vi "Boiler.vi"() -> ()   [LabVIEW 2013]
uses:
  Controls/Boiler Controls.ctl
  Controls/Boiler Simulation Controls.ctl
  Controls/Boiler Status Indicators.ctl
  Controls/Boiler Application Controls.ctl
  Controls/Boiler States.ctl
  Controls/Purge States.ctl
panel:
  in  "Stop":T1
  out "Boiler Status Indicators":T2 {"Time Count" format="%.2g"}
  in  "Boiler Simulation Controls":T3 {"Flame Sensor Value (%)" min=0.0 max=100.0 scale=0.0..100.0}
  in  "Boiler Controls":T4 {"Fuel Valve Position" min=0.0 max=100.0 scale=0.0..100.0 scale format="%.2f"}
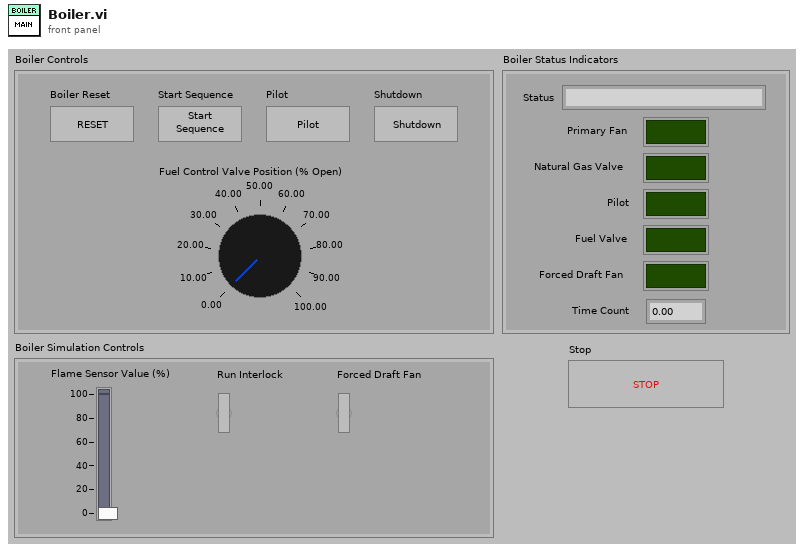
[diagram p1: front panel]
types:
  T1 = typedef "Boiler Application Controls.ctl" = bool
  T2 = typedef "Boiler Status Indicators.ctl" = cluster{"Status":string, "Primary Fan":bool, "Natural Gas Valve":bool, "Pilot":bool, "Fuel Valve":bool, "Forced Draft Fan":bool, "Time Count":dbl}
  T3 = typedef "Boiler Simulation Controls.ctl" = cluster{"Flame Sensor Value (%)":dbl, "Run Interlock":bool, "Forced Draft Fan":bool}
  T4 = typedef "Boiler Controls.ctl" = cluster{"Boiler Reset":bool, "Start Sequence":bool, "Pilot":bool, "Shutdown":bool, "Fuel Valve Position":dbl}
  T5 = typedef "Purge States.ctl" = enum16{"Pre-Purge", "Purge"}
  T6 = typedef "Boiler States.ctl" = enum16{"Initialize", "Main", "Reset Timeout", "Run Cont.", "Shutdown", "Stop"}
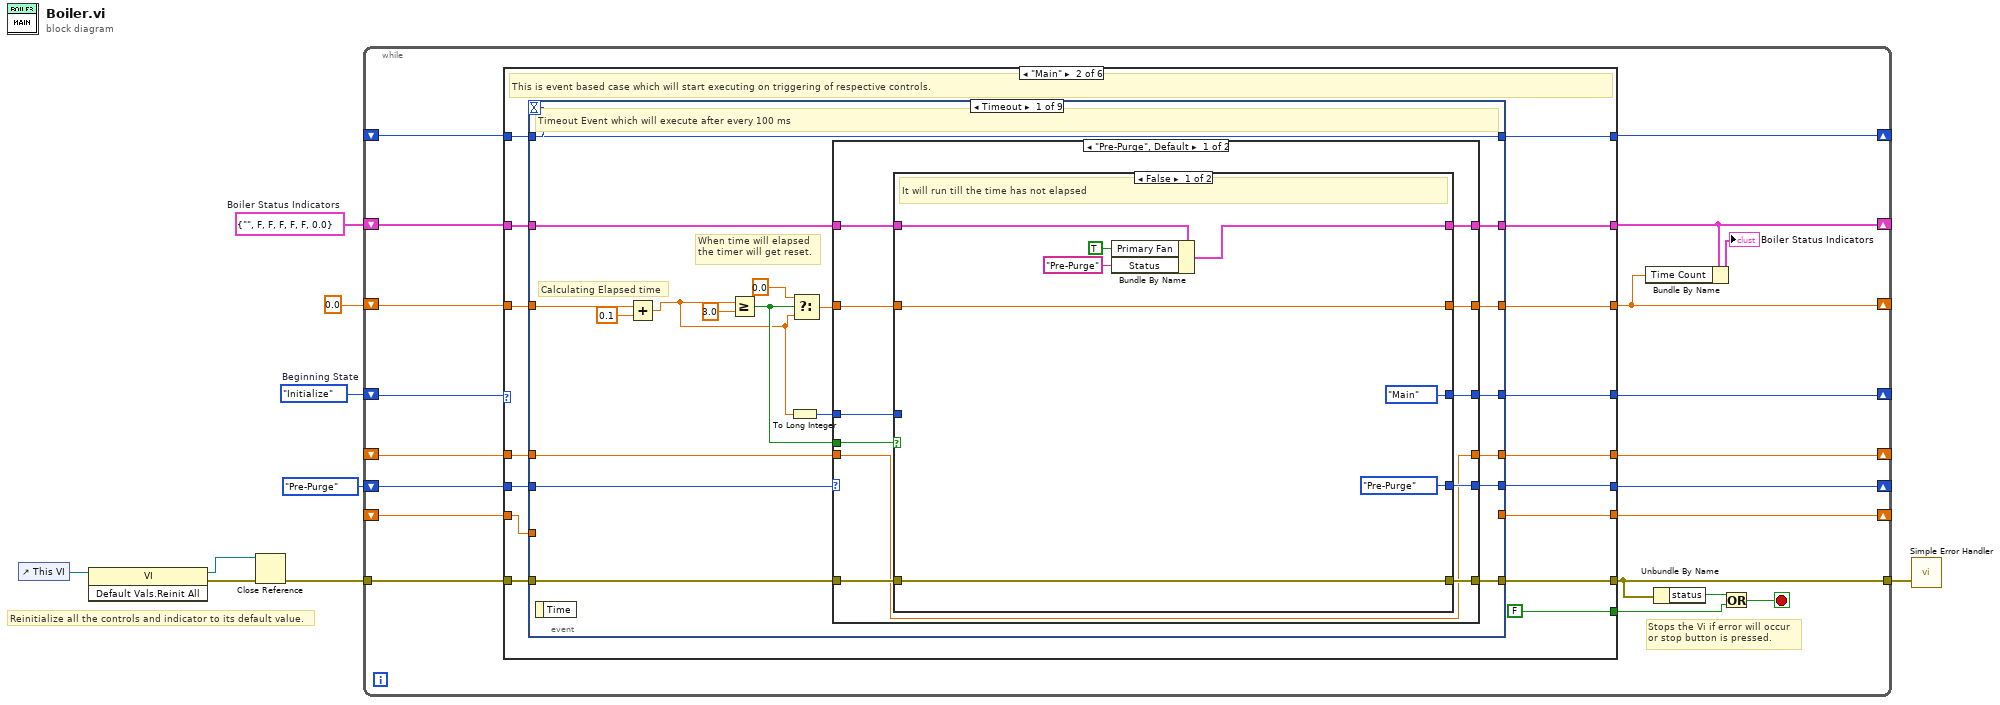
[diagram p0: block diagram]
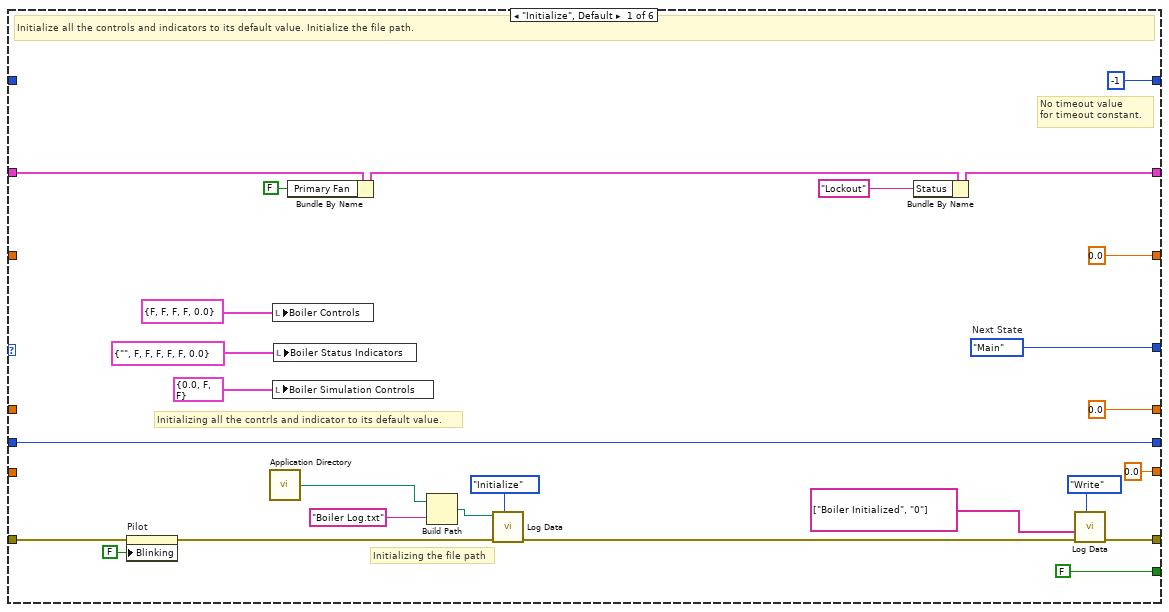
[diagram p2: hidden frame]
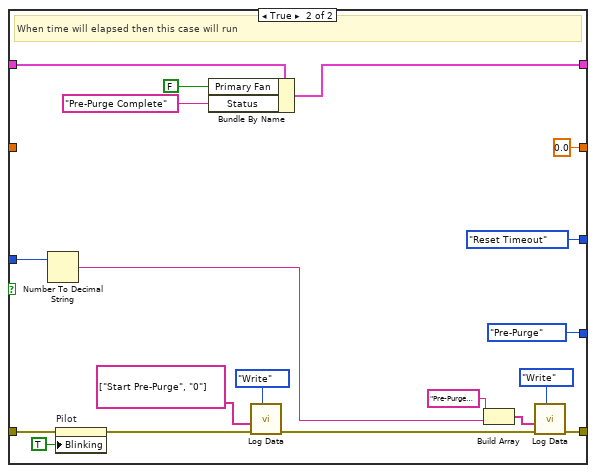
[diagram p3: hidden frame]
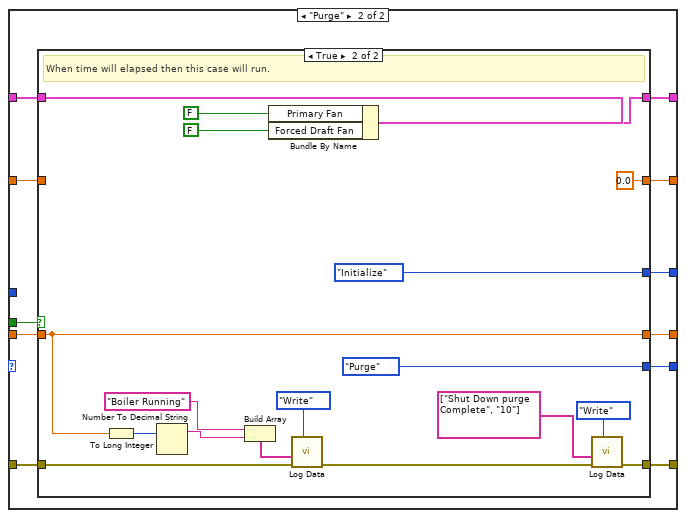
[diagram p4: hidden frame]
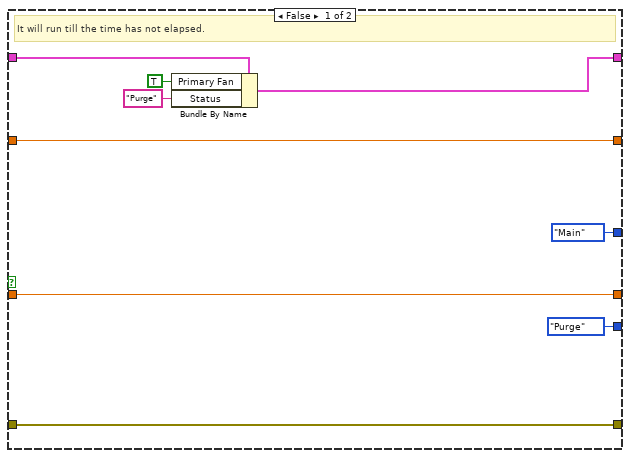
[diagram p5: hidden frame]
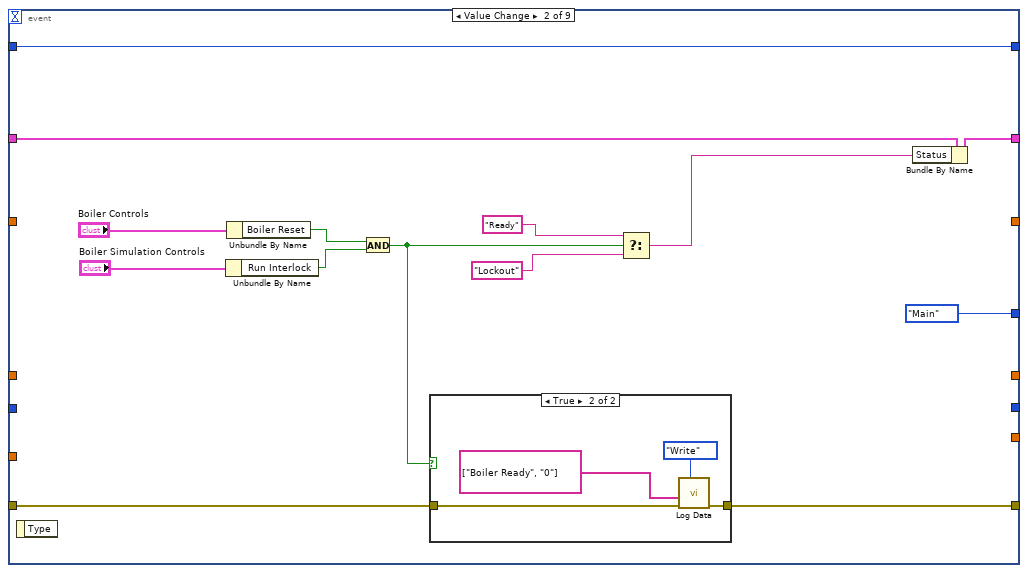
[diagram p6: hidden frame]
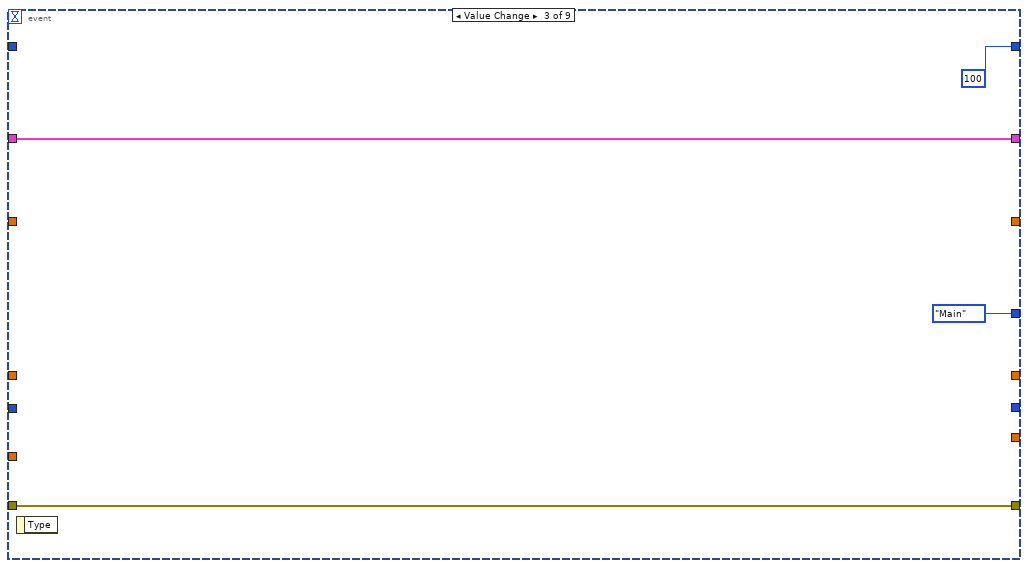
[diagram p8: hidden frame]
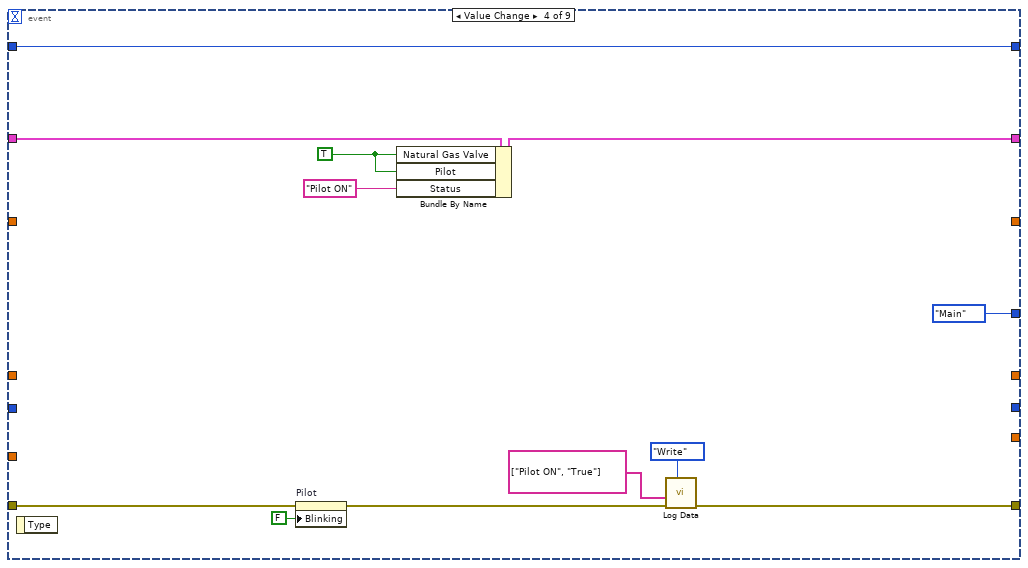
[diagram p9: hidden frame]
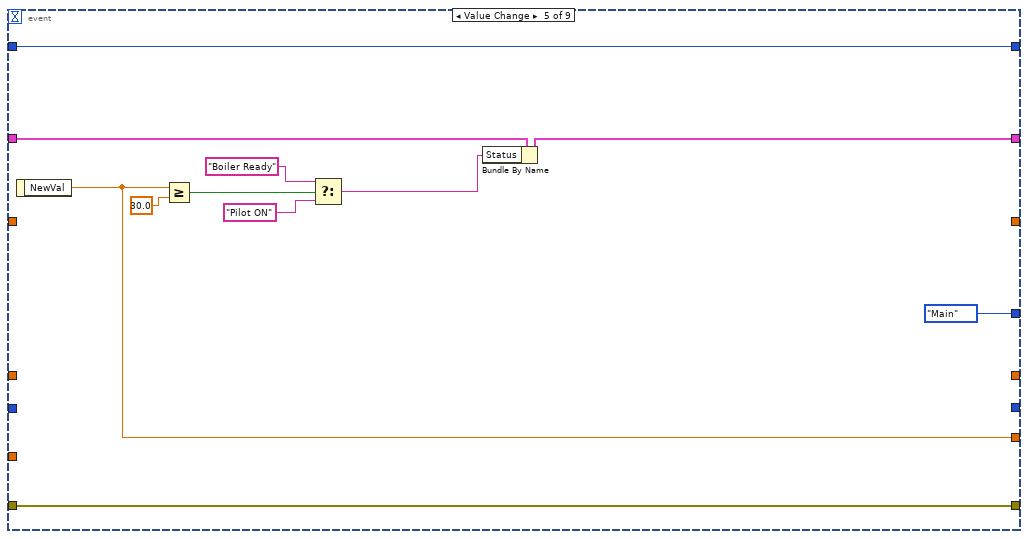
[diagram p10: hidden frame]
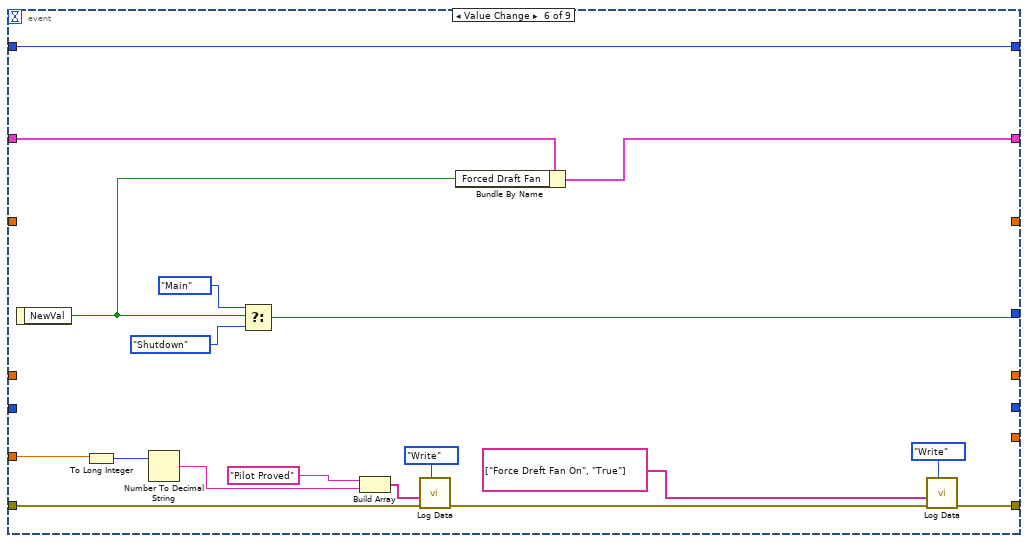
[diagram p11: hidden frame]
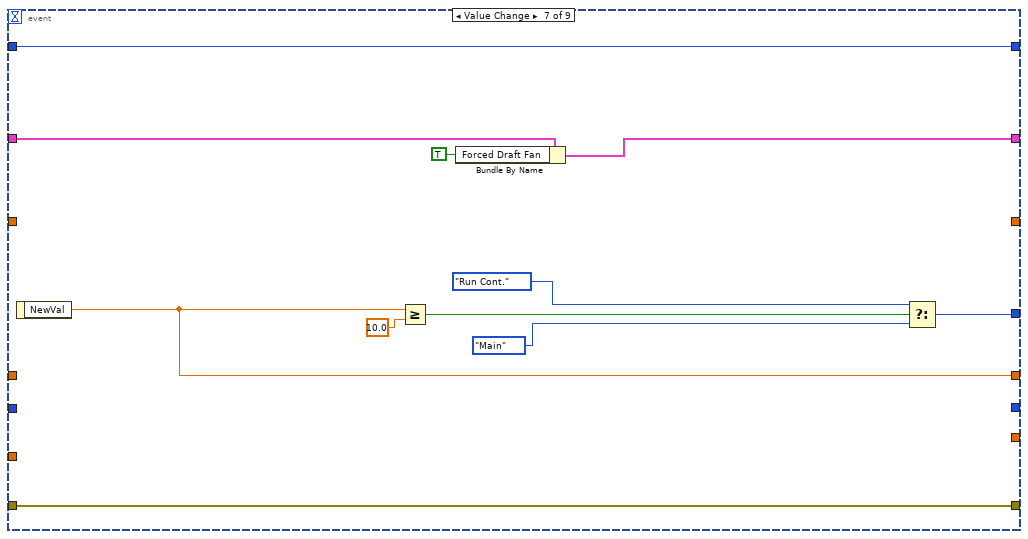
[diagram p12: hidden frame]
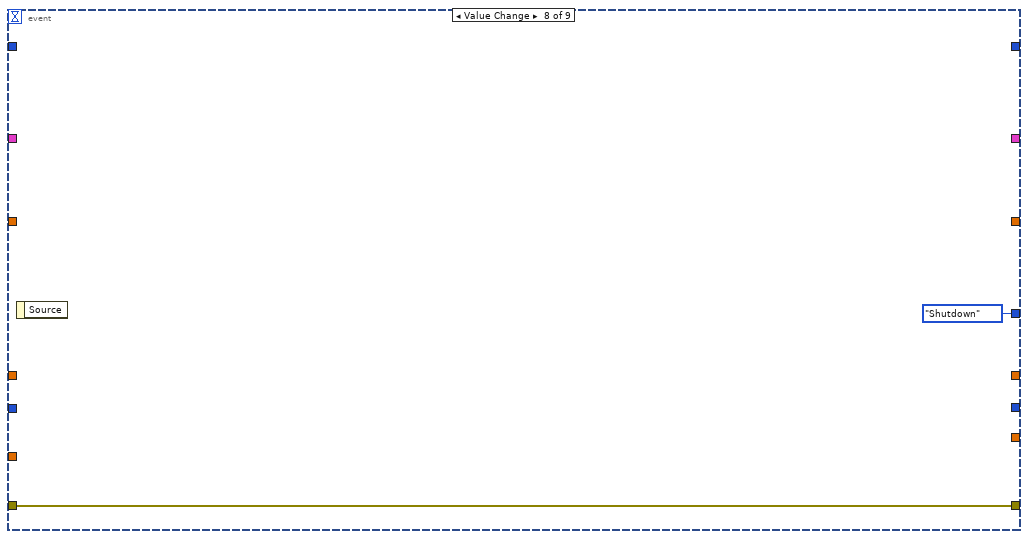
[diagram p13: hidden frame]
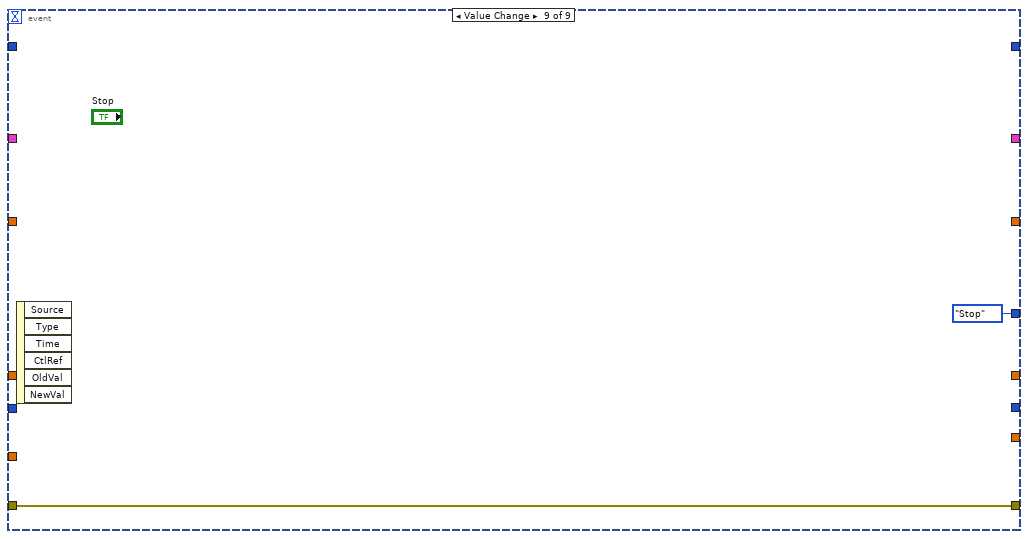
[diagram p14: hidden frame]
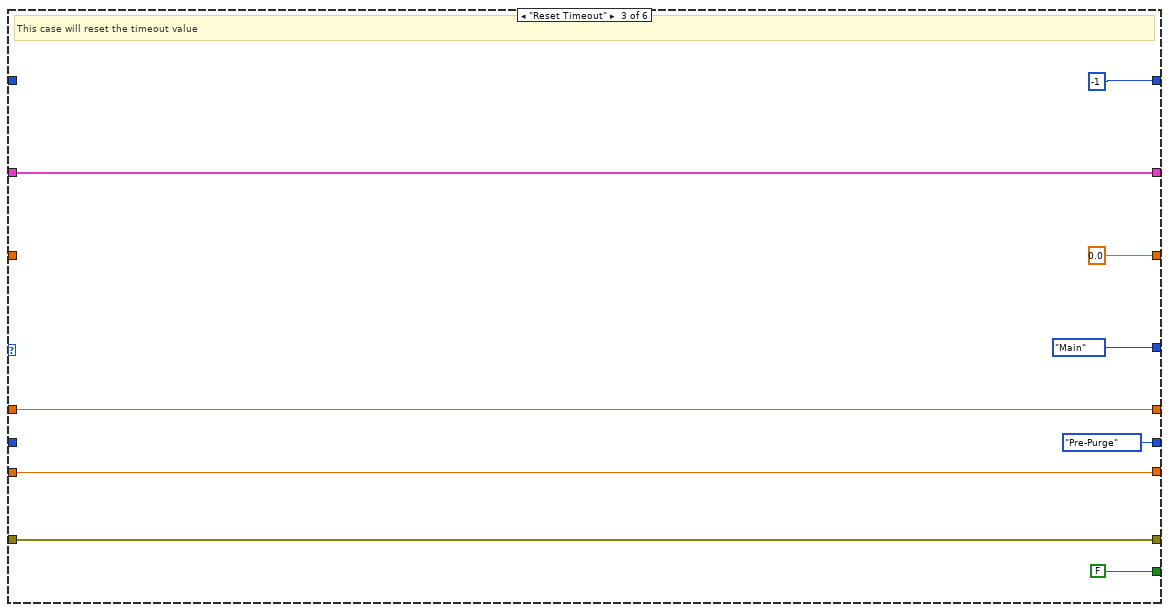
[diagram p15: hidden frame]
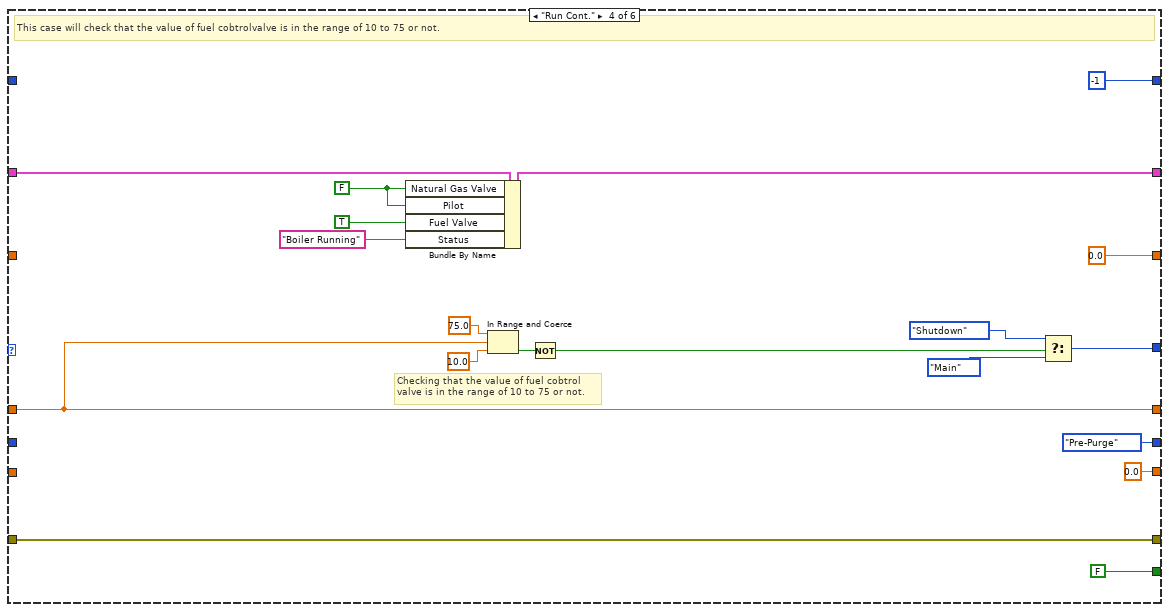
[diagram p16: hidden frame]
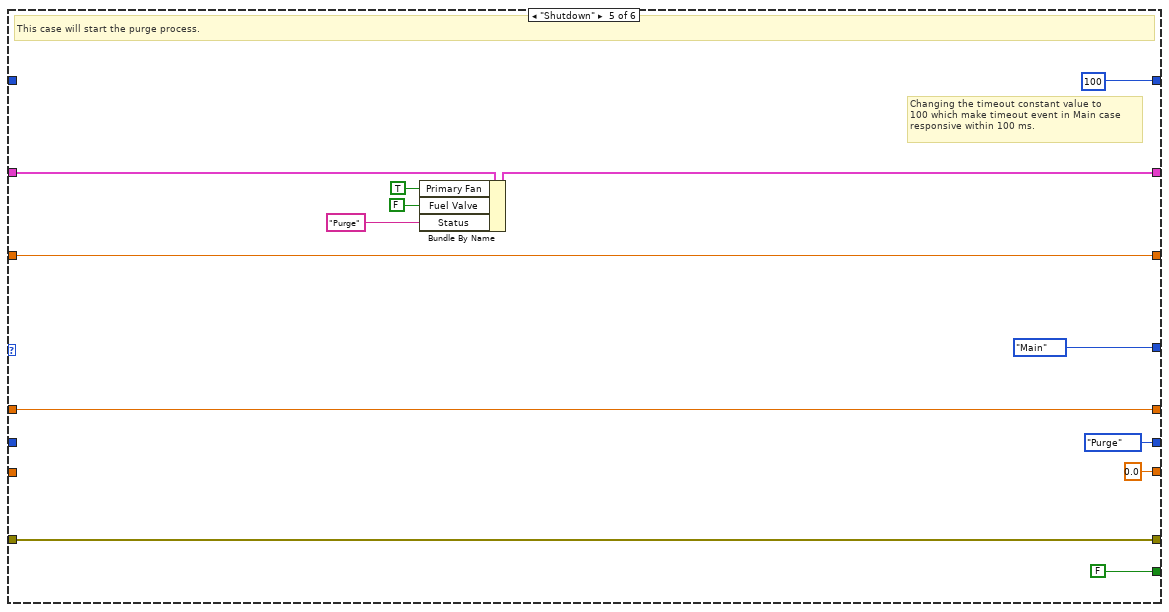
[diagram p17: hidden frame]
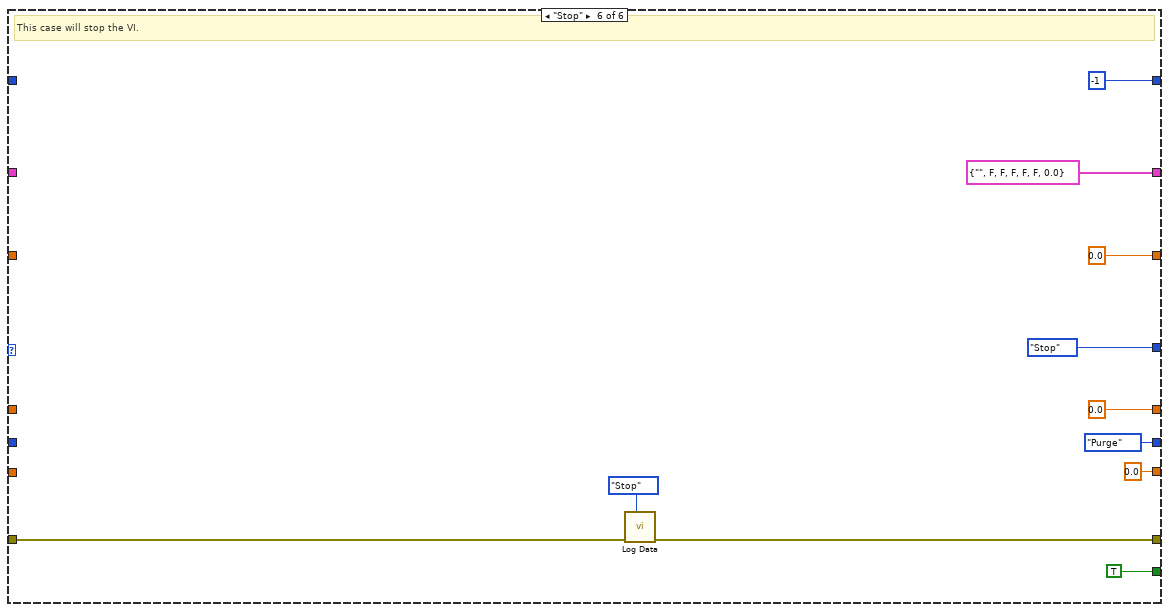
[diagram p18: hidden frame]
diagram:
  w3 = T2 {"Status"="", "Primary Fan"=FALSE, "Natural Gas Valve"=FALSE, "Pilot"=FALSE, "Fuel Valve"=FALSE, "Forced Draft Fan"=FALSE, "Time Count"=0.0}  # Boiler Status Indicators
  w9 = Boiler_States."Initialize"  # Beginning State
  # "Reinitialize all the controls and indicator to its default value."
  n1 = control-ref of="This VI"() -> (w8:refnum<vi>)
  n2 = invoke class="VI" method="Default Vals.Reinit All"(reference=w8) -> (reference out=w6:refnum<vi>, error out=w7:errorcluster)  [unwired: 2 in, 1 out]
  n3 = Close Reference(reference=w6, error in (no error)=w7) -> (error out=w5:errorcluster)
  n4 = while {
    shift-right: [w28] -> _
    shift-left: w9 -> [w29]
    tunnel: w5 -> [w27]
    tunnel: [w26] -> w4
    shift-right: [w22] -> _
    shift-left: _ -> [w19]
    shift-right: [w20] -> _
    shift-left: w3 -> [w21]
    shift-right: [w16] -> _
    shift-left: 0.0 -> [w18]
    shift-right: [w15] -> _
    shift-left: _ -> [w14]
    shift-right: [w12] -> _
    shift-left: Purge_States."Pre-Purge" -> [w13]
    shift-right: [w11] -> _
    shift-left: _ -> [w10]
    stop <- w25 stop-if-true
    # "Stops the Vi if error will occur \nor stop button is pressed."
    n5 = case shown="\"Main\"" w29 {
      tunnel: [w55 w62 Boiler_States."Main" ("Next State") w261 Boiler_States."Main" ("Next State") Boiler_States."Stop" ("Next State")] -> w28
      tunnel: w27 -> [w45 w70 w247 w271 w276 w290]
      tunnel: [w33 w69 w247 w271 w276 w289] -> w26
      tunnel: [FALSE FALSE FALSE FALSE FALSE TRUE] -> w23
      tunnel: [-1 w68 -1 -1 100 -1] -> w22
      tunnel: [w47 w66 w253 w269 w284 T2 {"Status"="", "Primary Fan"=FALSE, "Natural Gas Valve"=FALSE, "Pilot"=FALSE, "Fuel Valve"=FALSE, "Forced Draft Fan"=FALSE, "Time Count"=0.0} ("Boiler Status Indicators")] -> w20
      tunnel: w21 -> [w50 w67 w253 w273 w286 _]
      tunnel: w19 -> [_ w65 _ _ _ _]
      tunnel: w18 -> [_ w64 _ _ w277 _]
      tunnel: [0.0 ("t") w63 0.0 ("t") 0.0 ("t") w277 0.0 ("t")] -> w16
      tunnel: [0.0 ("NewVal") w61 w249 w260 w274 0.0 ("NewVal")] -> w15
      tunnel: w14 -> [_ w56 w249 w260 w274 _]
      tunnel: w13 -> [w42 w60 _ _ _ _]
      tunnel: [w42 w59 Purge_States."Pre-Purge" Purge_States."Pre-Purge" Purge_States."Purge" Purge_States."Purge"] -> w12
      tunnel: [0.0 ("NewVal") w58 w246 0.0 ("NewVal") 0.0 ("NewVal") 0.0 ("NewVal")] -> w11
      tunnel: w10 -> [_ w57 w246 _ _ _]
      frame "Initialize", Default {
        w55 = Boiler_States."Main"  # Next State
        # "No timeout value \nfor timeout constant."
        # "Initializing the file path"
        # "Initializing all the contrls and indicator to its default value."
        # "Initialize all the controls and indicators to its default value. Initialize the file path."
        n6 = property on="Pilot" class="Bool (strict)"(error in=w45, "Blinking"=FALSE) -> (error out=w39:errorcluster)  [unwired: 1 in, 1 out]
        n7 = call <vilib>:"Application Directory.vi"() -> ("Application Directory"=w37:path)
        n8 = local write "Boiler Controls"(T4 {"Boiler Reset"=FALSE, "Start Sequence"=FALSE, "Pilot"=FALSE, "Shutdown"=FALSE, "Fuel Valve Position"=0.0} ("Boiler Controls")) -> ()
        n9 = local write "Boiler Simulation Controls"(T3 {"Flame Sensor Value (%)"=0.0, "Run Interlock"=FALSE, "Forced Draft Fan"=FALSE} ("Boiler Simulation Controls")) -> ()
        n10 = local write "Boiler Status Indicators"(T2 {"Status"="", "Primary Fan"=FALSE, "Natural Gas Valve"=FALSE, "Pilot"=FALSE, "Fuel Valve"=FALSE, "Forced Draft Fan"=FALSE, "Time Count"=0.0} ("Boiler Status Indicators")) -> ()
        n11 = Bundle By Name(cluster=w50, "Primary Fan"=FALSE) -> (w41:T2)
        n12 = Build Path(base path=w37, name or relative path="Boiler Log.txt") -> (appended path=w36:path)
        n13 = call "Log Data.vi"("Command"=enum16{"Initialize", "Write", "Stop"}."Initialize", "error in (no error)"=w39, "file path"=w36) -> ("error out"=w34:errorcluster)  [unwired: 8 in]
        n14 = Bundle By Name(cluster=w41, "Status"="Lockout") -> (w47:T2)
        n15 = call "Log Data.vi"("Command"=enum16{"Initialize", "Write", "Stop"}."Write", "error in (no error)"=w34, "Event Data"=string[] ["Boiler Initialized", "0"]) -> ("error out"=w33:errorcluster)  [unwired: 8 in]
      }
      frame "Main" {
        # "This is event based case which will start executing on triggering of respective controls."
        n16 = event shown="[0] Timeout" {
          selector: _ -> [_ _ _ _ _ _ _ _ _]
          dyn-events: _ -> [_ _ _ _ _ _ _ _ _]
          timeout: w65 -> [_ _ _ _ _ _ _ _ _]
          tunnel: w70 -> [w82 w168 w189 w198 w202 w217 w232 w242 w245]
          tunnel: [w81 w167 w189 w192 w202 w223 w232 w242 w245] -> w69
          tunnel: [w86 w172 100 w199 w204 w228 w238 _ _] -> w68
          tunnel: w67 -> [w80 w175 w188 w201 w210 w229 w240 _ _]
          tunnel: [w79 w174 w188 w196 w209 w230 w241 _ _] -> w66
          tunnel: w65 -> [w86 w172 _ w199 w204 w228 w238 _ _]
          tunnel: [w84 _ _ _ _ _ _ _ _] -> w63
          tunnel: w64 -> [w90 _ _ _ _ _ _ _ _]
          tunnel: [w78 Boiler_States."Main" ("Next State") Boiler_States."Main" ("Next State") Boiler_States."Main" ("Next State") Boiler_States."Main" ("Next State") w225 w233 Boiler_States."Shutdown" ("Next State") Boiler_States."Stop" ("Next State")] -> w62
          tunnel: [w72 _ _ _ _ _ w231 _ _] -> w61
          tunnel: w60 -> [w77 _ _ _ _ _ _ _ _]
          tunnel: [w76 _ _ _ _ _ _ _ _] -> w59
          tunnel: [_ _ _ _ w203 _ _ _ _] -> w58
          tunnel: w57 -> [_ _ _ _ _ w214 _ _ _]
          tunnel: w56 -> [w73 _ _ _ _ _ _ _ _]
          event Timeout {
            # "When time will elapsed \nthe timer will get reset."
            # "Calculating Elapsed time"
            # "Timeout Event which will execute after every 100 ms"
            n17 = event-data() -> ()  [unwired: 1 in, 1 out]
            n18 = Add(x=w90, y=0.1) -> (x+y=w75:dbl)
            n19 = Greater Or Equal?(x=w75, y=3.0) -> (x >= y?=w85:bool)
            n20 = To Long Integer(number=w75) -> (32bit integer=w74:i32)
            n21 = Select(t=0.0, s=w85, f=w75) -> (s? t:f=w83:dbl)
            n22 = case shown="\"Pre-Purge\", Default" w77 {
              tunnel: w85 -> [w101 w139]
              tunnel: [w100 w138] -> w84
              tunnel: w83 -> [w99 w137]
              tunnel: w82 -> [w98 w136]
              tunnel: [w97 w135] -> w81
              tunnel: w80 -> [w96 w134]
              tunnel: [w95 w133] -> w79
              tunnel: [w94 w132] -> w78
              tunnel: [w93 w131] -> w76
              tunnel: w74 -> [w92 _]
              tunnel: w73 -> [w91 w130]
              tunnel: [w91 w129] -> w72
              frame "Pre-Purge", Default {
                n23 = case shown="False" w101 {
                  tunnel: [w109 0.0 ("t")] -> w100
                  tunnel: w99 -> [w109 _]
                  tunnel: w98 -> [w102 w127]
                  tunnel: [w102 w119] -> w97
                  tunnel: w96 -> [w106 w123]
                  tunnel: [w105 w122] -> w95
                  tunnel: [Boiler_States."Main" ("Next State") Boiler_States."Reset Timeout" ("Next State")] -> w94
                  tunnel: [Purge_States."Pre-Purge" Purge_States."Pre-Purge"] -> w93
                  tunnel: w92 -> [_ w118]
                  frame False {
                    # "It will run till the time has not elapsed"
                    n24 = Bundle By Name(cluster=w106, "Primary Fan"=TRUE, "Status"="Pre-Purge") -> (w105:T2)
                  }
                  frame True {
                    # "When time will elapsed then this case will run"
                    n25 = Number To Decimal String(number=w118) -> (decimal integer string=w117:string)  [unwired: 1 in]
                    n26 = property on="Pilot" class="Bool (strict)"(error in=w127, "Blinking"=TRUE) -> (error out=w112:errorcluster)  [unwired: 1 in, 1 out]
                    n27 = Bundle By Name(cluster=w123, "Primary Fan"=FALSE, "Status"="Pre-Purge Complete") -> (w122:T2)
                    n28 = call "Log Data.vi"("Command"=enum16{"Initialize", "Write", "Stop"}."Write", "error in (no error)"=w112, "Event Data"=string[] ["Start Pre-Purge", "0"]) -> ("error out"=w111:errorcluster)  [unwired: 8 in]
                    n29 = Build Array("Pre-Purge Complete", w117) -> (w114:string[])
                    n30 = call "Log Data.vi"("Command"=enum16{"Initialize", "Write", "Stop"}."Write", "error in (no error)"=w111, "Event Data"=w114) -> ("error out"=w119:errorcluster)  [unwired: 8 in]
                  }
                }
              }
              frame "Purge" {
                # "Pre-Purge Case"
                n31 = case shown="True" w139 {
                  tunnel: [w148 0.0 ("t")] -> w138
                  tunnel: w137 -> [w148 _]
                  tunnel: w136 -> [w147 w151]
                  tunnel: [w147 w157] -> w135
                  tunnel: w134 -> [w144 w165]
                  tunnel: [w143 w162] -> w133
                  tunnel: [Boiler_States."Main" ("Next State") Boiler_States."Initialize" ("Next State")] -> w132
                  tunnel: [Purge_States."Purge" Purge_States."Purge"] -> w131
                  tunnel: w130 -> [w140 w149]
                  tunnel: [w140 w149] -> w129
                  frame False {
                    # "It will run till the time has not elapsed."
                    n32 = Bundle By Name(cluster=w144, "Primary Fan"=TRUE, "Status"="Purge") -> (w143:T2)
                  }
                  frame True {
                    # "When time will elapsed then this case will run."
                    n33 = To Long Integer(number=w149) -> (32bit integer=w156:i32)
                    n34 = Number To Decimal String(number=w156) -> (decimal integer string=w155:string)  [unwired: 1 in]
                    n35 = Build Array("Boiler Running", w155) -> (w153:string[])
                    n36 = Bundle By Name(cluster=w165, "Primary Fan"=FALSE, "Forced Draft Fan"=FALSE) -> (w162:T2)
                    n37 = call "Log Data.vi"("Command"=enum16{"Initialize", "Write", "Stop"}."Write", "error in (no error)"=w151, "Event Data"=w153) -> ("error out"=w150:errorcluster)  [unwired: 8 in]
                    n38 = call "Log Data.vi"("Command"=enum16{"Initialize", "Write", "Stop"}."Write", "error in (no error)"=w150, "Event Data"=string[] ["Shut Down purge Complete", "10"]) -> ("error out"=w157:errorcluster)  [unwired: 8 in]
                  }
                }
              }
            }
          }
          event Value Change {
            n39 = event-data() -> ()  [unwired: 1 in, 1 out]
            n40 = Unbundle By Name("Boiler Simulation Controls") -> ("Run Interlock"=w171:bool)
            n41 = Unbundle By Name("Boiler Controls") -> ("Boiler Reset"=w178:bool)
            n42 = And(x=w178, y=w171) -> (x .and. y?=w169:bool)
            n43 = case shown="True" w169 {
              tunnel: w168 -> [w181 w185]
              tunnel: [w181 w184] -> w167
              frame False {
              }
              frame True {
                n44 = call "Log Data.vi"("Command"=enum16{"Initialize", "Write", "Stop"}."Write", "error in (no error)"=w185, "Event Data"=string[] ["Boiler Ready", "0"]) -> ("error out"=w184:errorcluster)  [unwired: 8 in]
              }
            }
            n45 = Select(t="Ready", s=w169, f="Lockout") -> (s? t:f=w173:string)
            n46 = Bundle By Name(cluster=w175, "Status"=w173) -> (w174:T2)
          }
          event Value Change {
            n47 = event-data() -> ()  [unwired: 1 in, 1 out]
          }
          event Value Change {
            w195 = TRUE ("Natural Gas Valve")
            n48 = event-data() -> ()  [unwired: 1 in, 1 out]
            n49 = property on="Pilot" class="Bool (strict)"(error in=w198, "Blinking"=FALSE) -> (error out=w193:errorcluster)  [unwired: 1 in, 1 out]
            n50 = Bundle By Name(cluster=w201, "Natural Gas Valve"=w195, "Pilot"=w195, "Status"="Pilot ON") -> (w196:T2)
            n51 = call "Log Data.vi"("Command"=enum16{"Initialize", "Write", "Stop"}."Write", "error in (no error)"=w193, "Event Data"=string[] ["Pilot ON", "True"]) -> ("error out"=w192:errorcluster)  [unwired: 8 in]
          }
          event Value Change {
            n52 = event-data() -> ("NewVal"=w203:dbl)  [unwired: 1 in]
            n53 = Greater Or Equal?(x=w203, y=30.0) -> (x >= y?=w211:bool)
            n54 = Select(t="Boiler Ready", s=w211, f="Pilot ON") -> (s? t:f=w206:string)
            n55 = Bundle By Name(cluster=w210, "Status"=w206) -> (w209:T2)
          }
          event Value Change {
            n56 = event-data() -> ("NewVal"=w224:bool)  [unwired: 1 in]
            n57 = To Long Integer(number=w214) -> (32bit integer=w218:i32)
            n58 = Number To Decimal String(number=w218) -> (decimal integer string=w219:string)  [unwired: 1 in]
            n59 = Select(t=Boiler_States."Main" ("Next State"), s=w224, f=Boiler_States."Shutdown" ("Next State")) -> (s? t:f=w225:T6)
            n60 = Build Array("Pilot Proved", w219) -> (w215:string[])
            n61 = call "Log Data.vi"("Command"=enum16{"Initialize", "Write", "Stop"}."Write", "error in (no error)"=w217, "Event Data"=w215) -> ("error out"=w216:errorcluster)  [unwired: 8 in]
            n62 = Bundle By Name(cluster=w229, "Forced Draft Fan"=w224) -> (w230:T2)
            n63 = call "Log Data.vi"("Command"=enum16{"Initialize", "Write", "Stop"}."Write", "error in (no error)"=w216, "Event Data"=string[] ["Force Dreft Fan On", "True"]) -> ("error out"=w223:errorcluster)  [unwired: 8 in]
          }
          event Value Change {
            n64 = event-data() -> ("NewVal"=w231:dbl)  [unwired: 1 in]
            n65 = Greater Or Equal?(x=w231, y=10.0) -> (x >= y?=w236:bool)
            n66 = Bundle By Name(cluster=w240, "Forced Draft Fan"=TRUE) -> (w241:T2)
            n67 = Select(t=Boiler_States."Run Cont." ("Next State"), s=w236, f=Boiler_States."Main" ("Next State")) -> (s? t:f=w233:T6)
          }
          event Value Change {
            n68 = event-data() -> ()  [unwired: 1 in, 1 out]
          }
          event Value Change {
            n69 = event-data() -> ()  [unwired: 1 in, 6 out]
          }
        }
      }
      frame "Reset Timeout" {
        # "This case will reset the timeout value"
      }
      frame "Run Cont." {
        w268 = FALSE ("Natural Gas Valve")
        # "Checking that the value of fuel cobtrol\nvalve is in the range of 10 to 75 or not."
        # "This case will check that the value of fuel cobtrolvalve is in the range of 10 to 75 or not."
        n70 = Bundle By Name(cluster=w273, "Natural Gas Valve"=w268, "Pilot"=w268, "Fuel Valve"=TRUE, "Status"="Boiler Running") -> (w269:T2)
        n71 = In Range and Coerce(upper limit=75.0, x=w260, lower limit=10.0) -> (In Range?=w259:bool)  [unwired: 1 out]
        n72 = Not(x=w259) -> (.not. x?=w258:bool)
        n73 = Select(t=Boiler_States."Shutdown", s=w258, f=Boiler_States."Main" ("Next State")) -> (s? t:f=w261:T6)
      }
      frame "Shutdown" {
        # "Changing the timeout constant value to \n100 which make timeout event in Main case\nresponsive within 100 ms."
        # "This case will start the purge process."
        n74 = Bundle By Name(cluster=w286, "Primary Fan"=TRUE, "Fuel Valve"=FALSE, "Status"="Purge") -> (w284:T2)
      }
      frame "Stop" {
        # "This case will stop the VI."
        n75 = call "Log Data.vi"("Command"=enum16{"Initialize", "Write", "Stop"}."Stop", "error in (no error)"=w290) -> ("error out"=w289:errorcluster)  [unwired: 9 in]
      }
    }
    n76 = Bundle By Name(cluster=w20, "Time Count"=w16) -> (→"Boiler Status Indicators":T2)
    n77 = Unbundle By Name(w26) -> ("status"=w24:bool)
    n78 = Or(x=w24, y=w23) -> (x .or. y?=w25:bool)
  }
  n79 = call <vilib>:"Simple Error Handler.vi"("error in (no error)"=w4) -> ()  [unwired: 4 in, 5 out]
